vi "LibXML_GetContentV2.vi"(8 "error in":errorcluster, 9 "index":i32, 11 "xmlXPathObj":u32) -> (0 "error out":errorcluster, 2 "content":string="the piezo x axis via adwin analog out", 3 "xmlXPathObj out":u32)   [LabVIEW 2019, in "Tools.lvlib" / "LibXML.lvlib"]
doc: "Gets resolved content of XPathObj at index input."
uses:
  LibXML.lvlib
  Error Cluster From Error Code_subroutine.vi
  LibXML_GetNodeStrPtr.vi
  LibXML_GetNodeResolvedContentStrPointer.vi
  LibXML_GetStringLength.vi
  LibXML_CopyString.vi
  <vilib>/Utility/error.llb/Trim Whitespace.vi
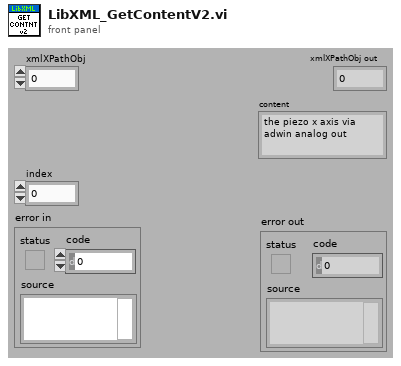
[diagram p1: front panel]
types:
  T1 = enum16{"NOP", "name", "content", "(resolved) content"}
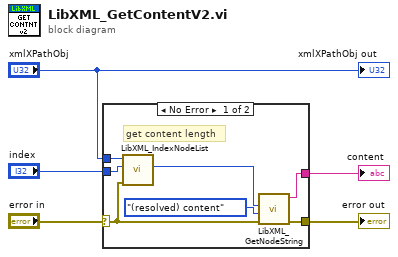
[diagram p0: block diagram]
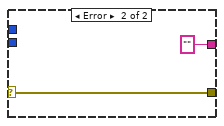
[diagram p2: hidden frame]
diagram:
  n1 = case shown="No Error" "error in" {
    selector: "error in" -> [w12 w14]
    tunnel: [w11 w14] -> w5
    tunnel: [w8 "" ("content")] -> w4
    tunnel: "xmlXPathObj" -> [w7 _]
    tunnel: "index" -> [w6 _]
    frame No Error {
      # "get content length"
      n2 = call "LibXML_IndexNodeList.vi"("error in"=w12, "index"=w6, "XPathObj"=w7) -> ("NodePtr"=w10:u32)  [unwired: 6 in, 2 out]
      n3 = call "LibXML_GetNodeString.vi"("error in"=w12, "type"=T1."(resolved) content", "node"=w10) -> ("error out"=w11:errorcluster, "lvstring"=w8:string)  [unwired: 7 in]
    }
    frame Error {
    }
  }
  "error out" <- w5
  "content" <- w4
  "xmlXPathObj out" <- "xmlXPathObj"
